vi "Read Channel Array.vi"(8 "error in":errorcluster, 10 "channels":refnum<class "Channel.lvclass">[](array[class]), 11 "digital output mode in":refnum<class "PWM Mode.lvclass">) -> (0 "error out":errorcluster, 2 "channel settings":T1[](array[typedef]), 3 "digital output mode out":refnum<class "PWM Mode.lvclass">)   [LabVIEW 2017, in "Scan Engine Scripting.lvlib" / "PWM Mode.lvclass"]
uses:
  PWM Mode.lvclass
  Channel Classes/Channel/Channel.lvclass
  Controls/pwm channel settings.ctl
  Channel Classes/PWM Output Channel/Frequency.ctl
  Channel Classes/PWM Output Channel/PWM Output Channel.lvclass
  Scan Engine Scripting.lvlib
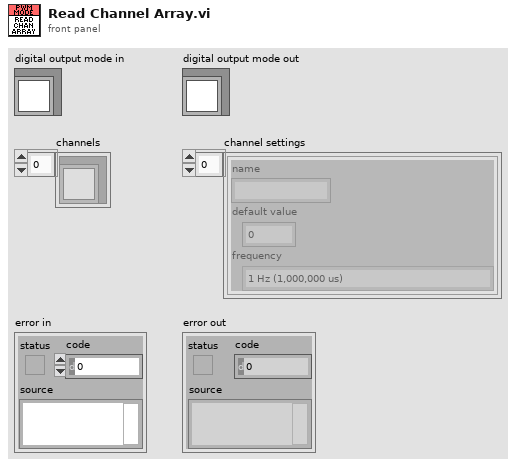
[diagram p1: front panel]
types:
  T1 = typedef "Scan Engine Scripting.lvlib/pwm channel settings.ctl" = cluster{"name":string, "default value":dbl, "frequency":T2}
  T2 = typedef "Scan Engine Scripting.lvlib/PWM Output Channel.lvclass/Frequency.ctl" = enum16{"1 Hz (1,000,000 us)", "50 Hz (20,000 us)", "250 Hz (4,000 us)", "500 Hz (2,000 us)", "1 kHz (1,000 us)", "5 kHz (200 us)", "10 kHz (100 us)", "20 kHz (50 us)"}
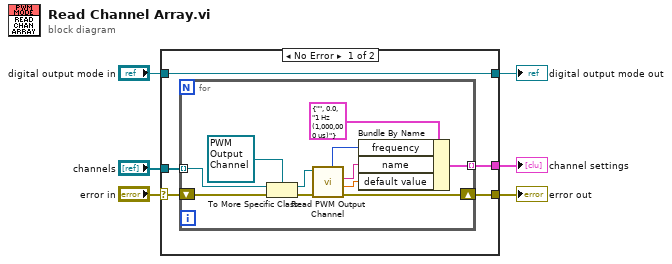
[diagram p0: block diagram]
diagram:
  n1 = case shown="No Error" "error in" {
    selector: "error in" -> [w9 w24]
    tunnel: [w8 w24] -> w5
    tunnel: [w11 w23] -> w3
    tunnel: "digital output mode in" -> [w11 w23]
    tunnel: "channels" -> [w10 _]
    tunnel: [w7 _] -> w1
    frame No Error {
      n2 = for {
        tunnel: w10 -> [w19] mode=indexing
        tunnel: [w21] -> w7 mode=indexing
        shift-right: [w18] -> w8
        shift-left: w9 -> [w20]
        n3 = To More Specific Class(target class=refnum<class "PWM Output Channel.lvclass"> refnum ("Scan Engine Scripting.lvlib:PWM Output Channel.lvclass"), reference=w19, error in=w20) -> (specific class reference=w13:refnum<class "PWM Output Channel.lvclass">, error out=w17:errorcluster)
        n4 = call "Read PWM Output Channel.vi"("error in"=w17, "PWM channel in"=w13) -> ("error out"=w18:errorcluster, "default value"=w15:dbl, "name"=w16:string, "frequency"=w12:T2)  [unwired: 4 in, 2 out]
        n5 = Bundle By Name(cluster=T1 {"name"="", "default value"=0.0, "frequency"=enum."1 Hz (1,000,000 us)"} ("channel settings"), "frequency"=w12, "name"=w16, "default value"=w15) -> (w21:T1)
      }
    }
    frame Error {
    }
  }
  "error out" <- w5
  "digital output mode out" <- w3
  "channel settings" <- w1
